vi "chooseKeeperPlay.vi"(8 "error in (no error)":errorcluster, 11 "Game in":refnum<class "Game.lvclass">) -> (0 "error out":errorcluster, 3 "Game out":refnum<class "Game.lvclass">)   [LabVIEW 2021, in "Game.lvclass"]
uses:
  Game.lvclass
  Team_class/KeeperPlay.ctl
  Game.lvclass/Game.ctl
  Team_class/Team.lvclass/Team.ctl
  HaltPlay_class/HaltPlay.lvclass
  ZigZagPlay_class/ZigZagPlay.lvclass
  BallPlacementPlay_class/BallPlacementPlay.lvclass
  Playbook_class/Playbook.lvclass/Playbook.ctl
  TestPlay_class/TestPlay.lvclass
  TimeoutPlay_class/TimeoutPlay.lvclass
  Playbook_class/Read keeper_plays.vi
  Read Referee.vi
  Read KeeperTeam.vi
  Team_class/Read KeeperPlay.vi
  Read AllyRef.vi
  Team_class/Write KeeperPlay.vi
  Write AllyRef.vi
  Write KeeperTeam.vi
  Ally_class/Ally.lvclass
  D:/RoboIme/horie/SSL_AI/Team_class/Team.lvclass
  Playbook_class/Playbook.lvclass
  Play_class/Play.lvclass
  KeeperPlay_class/KeeperPlay.lvclass
  GoToPlay_class/GoToPlay.lvclass
  BallPlacementAllyPlay_class/BallPlacementAllyPlay.lvclass
  SimpleBallPlacementAllyPlay_class/SimpleBallPlacementAllyPlay.lvclass
  Referee_class/Referee.lvclass
panel:
  in  "keeperPlaysEnum\n(default control)":T1[](array[typedef])=[enum."TestPlay", enum."Halt", enum."Timeout", enum."ZigZag", enum."BallPlacementEnemy", enum."BallPlacementAlly", enum."SimpleBallPlacementAlly", enum."KeeperPlay"]
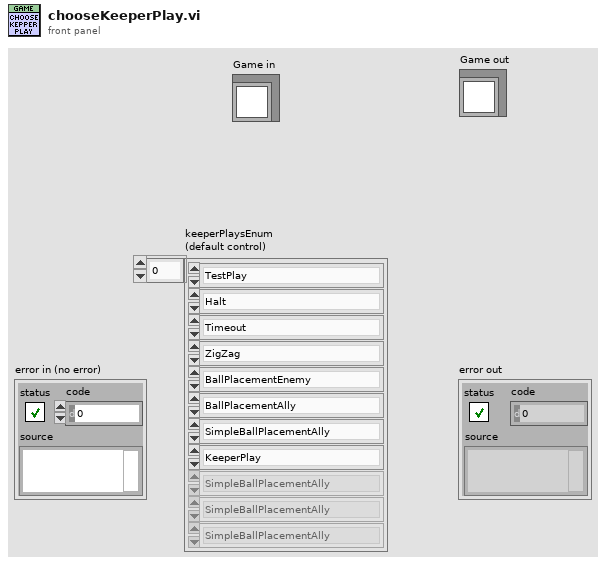
[diagram p1: front panel]
types:
  T1 = typedef "KeeperPlay.ctl" = enum16{"SimpleBallPlacementAlly", "BallPlacementAlly", "BallPlacementEnemy", "ZigZag", "Goto", "NormalGame", "KeeperPlay", "Halt", "Timeout", "PenaltyEnemy", "TestPlay"}
  T2 = typedef "keeper_plays.ctl" = cluster{"Play":refnum<class "Play.lvclass">, "TestPlay":refnum<class "TestPlay.lvclass">, "HaltPlay":refnum<class "HaltPlay.lvclass">, "KeeperPlay":refnum<class "KeeperPlay.lvclass">, "TimeoutPlay":refnum<class "TimeoutPlay.lvclass">, "ZigZagPlay":refnum<class "ZigZagPlay.lvclass">, "GoToPlay":refnum<class "GoToPlay.lvclass">, "BallPlacementPlay":refnum<class "BallPlacementPlay.lvclass">, "BallPlacementAllyPlay":refnum<class "BallPlacementAllyPlay.lvclass">, "SimpleBallPlacementAllyPlay":refnum<class "SimpleBallPlacementAllyPlay.lvclass">}
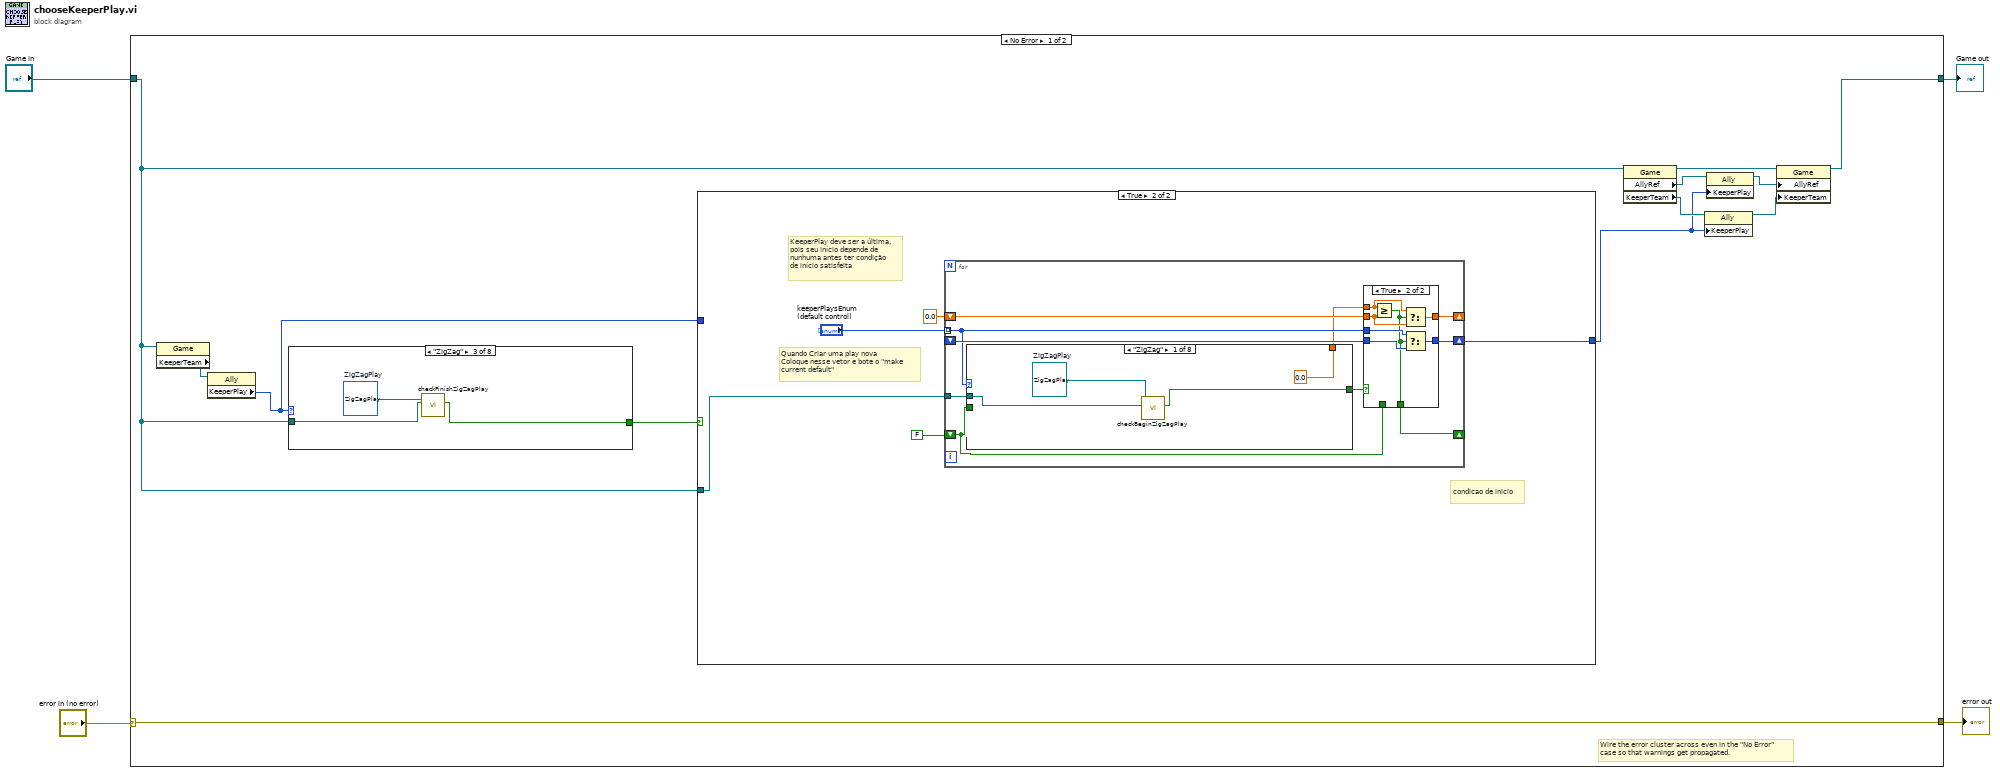
[diagram p0: block diagram]
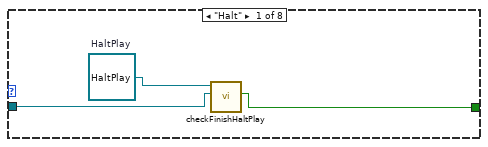
[diagram p2: hidden frame]
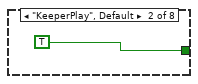
[diagram p3: hidden frame]
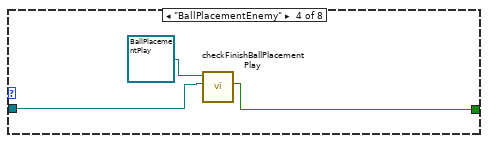
[diagram p4: hidden frame]
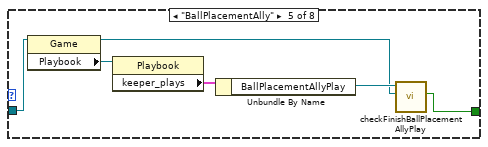
[diagram p5: hidden frame]
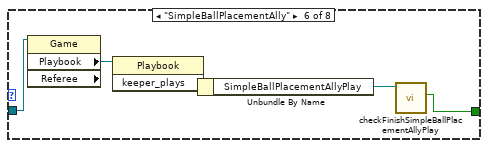
[diagram p6: hidden frame]
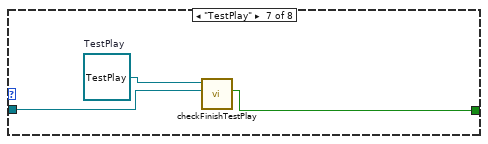
[diagram p7: hidden frame]
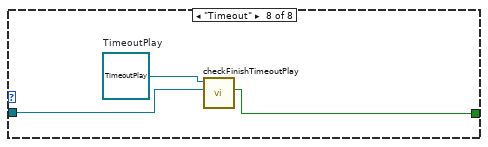
[diagram p8: hidden frame]
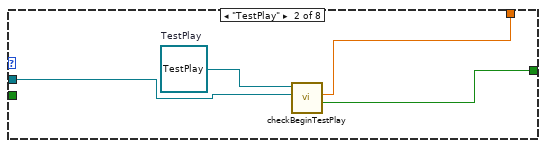
[diagram p10: hidden frame]
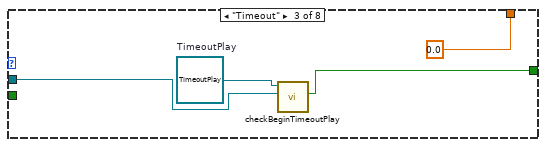
[diagram p11: hidden frame]
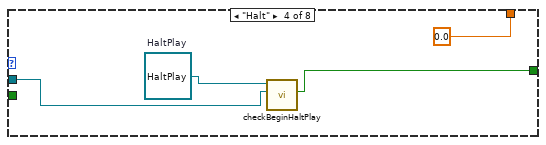
[diagram p12: hidden frame]
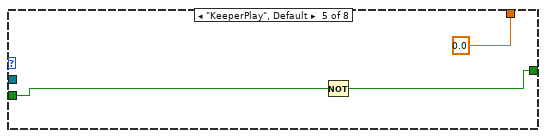
[diagram p13: hidden frame]
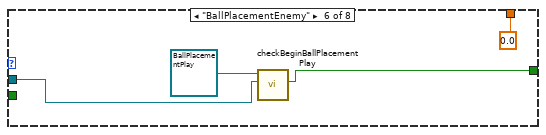
[diagram p14: hidden frame]
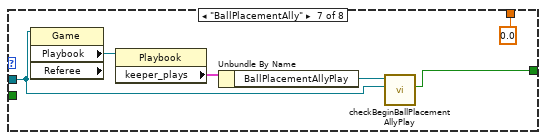
[diagram p15: hidden frame]
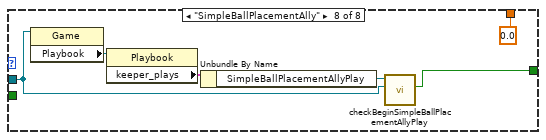
[diagram p16: hidden frame]
diagram:
  n1 = case shown="No Error" "error in (no error)" {
    selector: "error in (no error)" -> [w16 w106]
    tunnel: [w16 w106] -> w3
    tunnel: [w14 w105] -> w1
    tunnel: "Game in" -> [w8 w105]
    frame No Error {
      # "Wire the error cluster across even in the \"No Error\"\ncase so that warnings get propagated."
      n2 = property class="Game"(reference=w8) -> ("KeeperTeam"=w13:refnum<class "Ally.lvclass">)  [unwired: 1 in, 2 out]
      n3 = property class="Ally"(reference=w13) -> ("KeeperPlay"=w11:T1)  [unwired: 1 in, 2 out]
      n4 = case shown="\"ZigZag\"" w11 {
        tunnel: [w17 TRUE w21 w24 w29 w33 w38 w41] -> w12
        tunnel: w8 -> [w18 _ w22 w25 w28 w34 w39 w42]
        frame "Halt" {
          w19 = refnum<class "HaltPlay.lvclass"> refnum  # HaltPlay
          n5 = call "checkFinishHaltPlay.vi"("Game"=w18, "HaltPlay in"=w19) -> ("Boolean"=w17:bool)  [unwired: 7 in, 2 out]
        }
        frame "KeeperPlay", Default {
        }
        frame "ZigZag" {
          w23 = refnum<class "ZigZagPlay.lvclass"> refnum  # ZigZagPlay
          n6 = call "checkFinishZigZagPlay.vi"("Game"=w22, "ZigZagPlay in"=w23) -> ("Boolean"=w21:bool)  [unwired: 7 in, 2 out]
        }
        frame "BallPlacementEnemy" {
          n7 = call "checkFinishBallPlacementPlay.vi"("Game in"=w25, "BallPlacementPlay in"=refnum<class "BallPlacementPlay.lvclass"> refnum) -> ("finish?"=w24:bool)  [unwired: 7 in, 2 out]
        }
        frame "BallPlacementAlly" {
          n8 = property class="Game"(reference=w28) -> (reference out=w27:refnum<class "Game.lvclass">, "Playbook"=w31:refnum<class "Playbook.lvclass">)  [unwired: 1 in, 1 out]
          n9 = property class="Playbook"(reference=w31) -> ("keeper_plays"=w32:T2)  [unwired: 1 in, 2 out]
          n10 = Unbundle By Name(w32) -> ("BallPlacementAllyPlay"=w30:refnum<class "BallPlacementAllyPlay.lvclass">)
          n11 = call "checkFinishBallPlacementAllyPlay.vi"("Game"=w27, "BallPlacementAllyPlay in"=w30) -> ("finishBallPlacementAlly"=w29:bool)  [unwired: 7 in, 2 out]
        }
        frame "SimpleBallPlacementAlly" {
          n12 = property class="Game" props=["Playbook", "Referee"](reference=w34) -> ("Playbook"=w36:refnum<class "Playbook.lvclass">)  [unwired: 1 in, 3 out]
          n13 = property class="Playbook"(reference=w36) -> ("keeper_plays"=w37:T2)  [unwired: 1 in, 2 out]
          n14 = Unbundle By Name(w37) -> ("SimpleBallPlacementAllyPlay"=w35:refnum<class "SimpleBallPlacementAllyPlay.lvclass">)
          n15 = call "checkFinishSimpleBallPlacementAllyPlay.vi"("SimpleBallPlacementAllyPlay in"=w35) -> ("finish"=w33:bool)  [unwired: 8 in, 2 out]
        }
        frame "TestPlay" {
          w40 = refnum<class "TestPlay.lvclass"> refnum  # TestPlay
          n16 = call "checkFinishTestPlay.vi"("Game"=w39, "TestPlay in"=w40) -> ("Boolean"=w38:bool)  [unwired: 7 in, 2 out]
        }
        frame "Timeout" {
          w43 = refnum<class "TimeoutPlay.lvclass"> refnum  # TimeoutPlay
          n17 = call "checkFinishTimeoutPlay.vi"("Game"=w42, "TimeoutPlay in"=w43) -> ("Finish Timeout?"=w41:bool)  [unwired: 7 in, 2 out]
        }
      }
      n18 = case shown="True" w12 {
        tunnel: [w44 w48] -> w5
        tunnel: w11 -> [w44 _]
        tunnel: w8 -> [_ w46]
        frame False {
        }
        frame True {
          # "Quando Criar uma play nova\nColoque nesse vetor e bote o \"make\ncurrent default\""
          # "KeeperPlay deve ser a última,\npois seu início depende de \nnunhuma antes ter condição\nde início satisfeita"
          # "condicao de inicio"
          n19 = for {
            tunnel: "keeperPlaysEnum\n(default control)" -> [w55] mode=indexing
            shift-right: [w58] -> _
            shift-left: 0.0 -> [w57]
            shift-right: [w56] -> w48
            shift-left: _ -> [w59]
            shift-right: [w52] -> _
            shift-left: FALSE -> [w51]
            tunnel: w46 -> [w50]
            n20 = case shown="\"ZigZag\"" w55 {
              tunnel: [w62 w66 w70 w74 w78 w81 w84 w90] -> w54
              tunnel: [0.0 w65 0.0 0.0 0.0 0.0 ("Score out") 0.0 ("Score out") 0.0 ("Score out")] -> w53
              tunnel: w51 -> [_ _ _ _ w77 _ _ _]
              tunnel: w50 -> [w60 w64 w68 w72 _ w79 w83 w89]
              frame "ZigZag" {
                w61 = refnum<class "ZigZagPlay.lvclass"> refnum  # ZigZagPlay
                n21 = call "checkBeginZigZagPlay.vi"("Game"=w60, "ZigZagPlay in"=w61) -> ("TestMode"=w62:bool)  [unwired: 7 in, 2 out]
              }
              frame "TestPlay" {
                w67 = refnum<class "TestPlay.lvclass"> refnum  # TestPlay
                n22 = call "checkBeginTestPlay.vi"("Game"=w64, "TestPlay in"=w67) -> ("Test"=w66:bool, "Score out"=w65:dbl)  [unwired: 6 in, 2 out]
              }
              frame "Timeout" {
                w71 = refnum<class "TimeoutPlay.lvclass"> refnum  # TimeoutPlay
                n23 = call "checkBeginTimeoutPlay.vi"("Game"=w68, "TimeoutPlay in"=w71) -> ("BeginTimeout?"=w70:bool)  [unwired: 7 in, 2 out]
              }
              frame "Halt" {
                w75 = refnum<class "HaltPlay.lvclass"> refnum  # HaltPlay
                n24 = call "checkBeginHaltPlay.vi"("Game"=w72, "HaltPlay in"=w75) -> ("Boolean"=w74:bool)  [unwired: 7 in, 2 out]
              }
              frame "KeeperPlay", Default {
                n25 = Not(x=w77) -> (.not. x?=w78:bool)
              }
              frame "BallPlacementEnemy" {
                n26 = call "checkBeginBallPlacementPlay.vi"("Game in"=w79, "BallPlacementPlay in"=refnum<class "BallPlacementPlay.lvclass"> refnum) -> ("begin?"=w81:bool)  [unwired: 7 in, 2 out]
              }
              frame "BallPlacementAlly" {
                n27 = property class="Game" props=["Playbook", "Referee"](reference=w83) -> ("Playbook"=w87:refnum<class "Playbook.lvclass">)  [unwired: 1 in, 3 out]
                n28 = property class="Playbook"(reference=w87) -> ("keeper_plays"=w88:T2)  [unwired: 1 in, 2 out]
                n29 = Unbundle By Name(w88) -> ("BallPlacementAllyPlay"=w86:refnum<class "BallPlacementAllyPlay.lvclass">)
                n30 = call "checkBeginBallPlacementAllyPlay.vi"("Game"=w83, "BallPlacementAllyPlay in"=w86) -> ("BeginBallPlacementAlly"=w84:bool)  [unwired: 7 in, 2 out]
              }
              frame "SimpleBallPlacementAlly" {
                n31 = property class="Game"(reference=w89) -> ("Playbook"=w93:refnum<class "Playbook.lvclass">)  [unwired: 1 in, 2 out]
                n32 = property class="Playbook"(reference=w93) -> ("keeper_plays"=w94:T2)  [unwired: 1 in, 2 out]
                n33 = Unbundle By Name(w94) -> ("SimpleBallPlacementAllyPlay"=w92:refnum<class "SimpleBallPlacementAllyPlay.lvclass">)
                n34 = call "checkBeginSimpleBallPlacementAllyPlay.vi"("Game"=w89, "SimpleBallPlacementAllyPlay in"=w92) -> ("begin"=w90:bool)  [unwired: 7 in, 2 out]
              }
            }
            n35 = case shown="True" w54 {
              tunnel: w59 -> [w96 w101]
              tunnel: [w97 w104] -> w58
              tunnel: w57 -> [w97 w100]
              tunnel: w55 -> [_ w102]
              tunnel: [w96 w103] -> w56
              tunnel: w53 -> [_ w99]
              tunnel: [w95 w98] -> w52
              tunnel: w51 -> [w95 _]
              frame False {
              }
              frame True {
                n36 = Greater Or Equal?(x=w99, y=w100) -> (x >= y?=w98:bool)
                n37 = Select(t=w99, s=w98, f=w100) -> (s? t:f=w104:dbl)
                n38 = Select(t=w102, s=w98, f=w101) -> (s? t:f=w103:T1)
              }
            }
          }
        }
      }
      n39 = property class="Game"(reference=w8) -> (reference out=w15:refnum<class "Game.lvclass">, "AllyRef"=w7:refnum<class "Ally.lvclass">, "KeeperTeam"=w10:refnum<class "Ally.lvclass">)  [unwired: 1 in, 1 out]
      n40 = property class="Ally"(reference=w10, "KeeperPlay"=w5) -> (reference out=w9:refnum<class "Ally.lvclass">)  [unwired: 1 in, 1 out]
      n41 = property class="Ally"(reference=w7, "KeeperPlay"=w5) -> (reference out=w6:refnum<class "Ally.lvclass">)  [unwired: 1 in, 1 out]
      n42 = property class="Game"(reference=w15, "AllyRef"=w6, "KeeperTeam"=w9) -> (reference out=w14:refnum<class "Game.lvclass">)  [unwired: 1 in, 1 out]
    }
    frame Error {
    }
  }
  "error out" <- w3
  "Game out" <- w1
